vi "signalAccumulate.vi"() -> ()   [LabVIEW 2018]
panel:
  out "yArray":sgl[](array[numeric])
  out "xArray":dbl[](array[numeric])
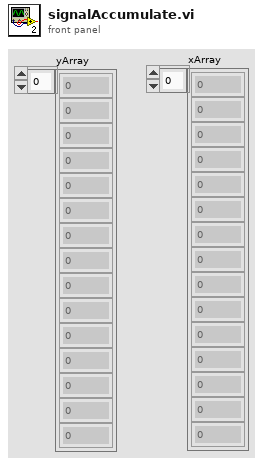
[diagram p1: front panel]
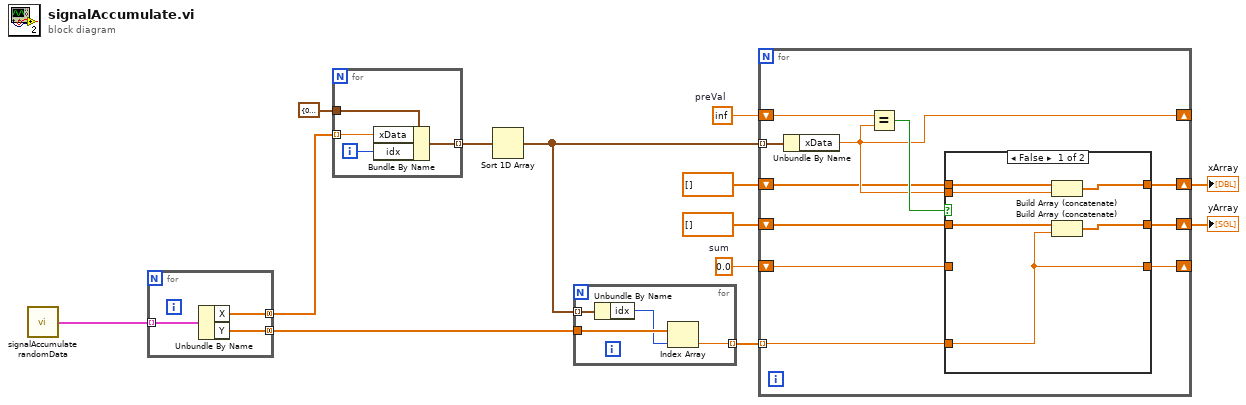
[diagram p0: block diagram]
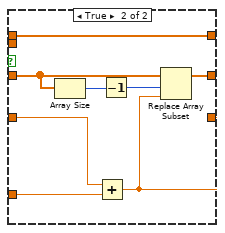
[diagram p2: hidden frame]
diagram:
  w7 = sgl 0.0  # sum
  w8 = inf  # preVal
  n1 = call "signalAccumulate randomData.vi"() -> ("Data"=w13:cluster{"X":dbl[], "Y":sgl[]}[])
  n2 = for {
    tunnel: w13 -> [w16] mode=indexing
    tunnel: [w15] -> w12 mode=concatenating
    tunnel: [w14] -> w4 mode=concatenating
    n3 = Unbundle By Name(w16) -> ("X"=w15:dbl[], "Y"=w14:sgl[])
  }
  n4 = for {
    tunnel: w12 -> [w19] mode=indexing
    tunnel: cluster{"xData":dbl, "idx":i32} {"xData"=0.0, "idx"=0} -> [w20]
    tunnel: [w17] -> w10 mode=indexing
    i -> [w18]
    n5 = Bundle By Name(cluster=w20, "xData"=w19, "idx"=w18) -> (w17:cluster{"xData":dbl, "idx":i32})
  }
  n6 = Sort 1D Array(array=w10) -> (sorted array=w9:cluster{"xData":dbl, "idx":i32}[])
  n7 = for {
    tunnel: w9 -> [w24] mode=indexing
    tunnel: w4 -> [w23]
    tunnel: [w21] -> w3 mode=indexing
    n8 = Unbundle By Name(w24) -> ("idx"=w22:i32)
    n9 = Index Array(array=w23, index=w22) -> (element=w21:sgl)
  }
  n10 = for {
    tunnel: w9 -> [w35] mode=indexing
    shift-right: [w27] -> _
    shift-left: w8 -> [w34]
    tunnel: w3 -> [w32] mode=indexing
    shift-right: [w30] -> w5
    shift-left: sgl[] [] -> [w31]
    shift-right: [w28] -> _
    shift-left: w7 -> [w29]
    shift-right: [w25] -> w6
    shift-left: dbl[] [] -> [w26]
    n11 = Unbundle By Name(w35) -> ("xData"=w27:dbl)
    n12 = Equal?(x=w34, y=w27) -> (x = y?=w33:bool)
    n13 = case shown="False" w33 {
      tunnel: w32 -> [w39 w49]
      tunnel: w31 -> [w41 w46]
      tunnel: [w40 w47] -> w30
      tunnel: w29 -> [_ w48]
      tunnel: [w39 w44] -> w28
      tunnel: w27 -> [w37 _]
      tunnel: w26 -> [w38 w43]
      tunnel: [w36 w43] -> w25
      frame False {
        n14 = Build Array (concatenate)(w38, w37) -> (w36:dbl[])
        n15 = Build Array (concatenate)(w41, w39) -> (w40:sgl[])
      }
      frame True {
        n16 = Array Size(array=w46) -> (size(s)=w45:i32)
        n17 = Add(x=w48, y=w49) -> (x+y=w44:sgl)
        n18 = Decrement(x=w45) -> (x-1=w42:i32)
        n19 = Replace Array Subset(array=w46, new element=w44, index=w42) -> (w47:sgl[])
      }
    }
  }
  "xArray" <- w6
  "yArray" <- w5
